vi "SetTilesByString.vi"(8 "error in (no error)":errorcluster, 9 "Position":T1, 10 "TileStrings":string[][](array[string]), 11 "TilesQueue":refnum<queue>) -> (0 "error out":errorcluster, 3 "TilesQueue out":refnum<queue>)   [LabVIEW 2019, in "RT_Game.lvlib" / "Engine.lvclass"]
uses:
  Engine.lvclass
  Game/Coordinate.ctl
  MessageCluster.ctl
  SetTilesByStringData.ctl
  Game/Game.lvclass
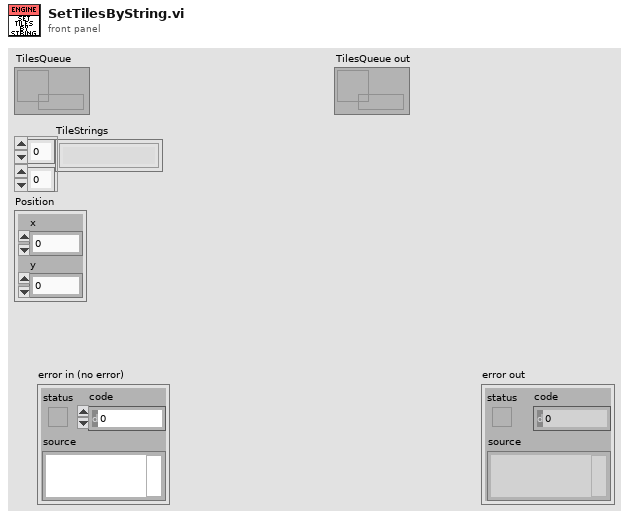
[diagram p1: front panel]
types:
  T1 = typedef "RT_Game.lvlib/Game.lvclass/Coordinate.ctl" = cluster{"x":dbl, "y":dbl}
  T2 = typedef "RT_Game.lvlib/Engine.lvclass/MessageCluster.ctl" = cluster{"Message":string, "Data":variant}
  T3 = typedef "RT_Game.lvlib/Engine.lvclass/SetTilesByStringData.ctl" = cluster{"TileStrings":string[][], "Position":T1}
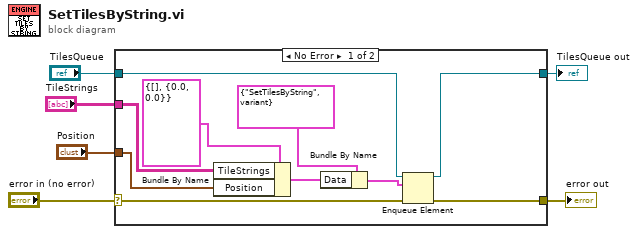
[diagram p0: block diagram]
diagram:
  n1 = case shown="No Error" "error in (no error)" {
    selector: "error in (no error)" -> [w11 w18]
    tunnel: [w12 w18] -> w5
    tunnel: "TileStrings" -> [w10 _]
    tunnel: "Position" -> [w9 _]
    tunnel: "TilesQueue" -> [w8 w17]
    tunnel: [w7 w17] -> w1
    frame No Error {
      n2 = Bundle By Name(cluster=T3 {"TileStrings"=[], "Position"={"x"=0.0, "y"=0.0}} ("SetTilesByStringData"), "TileStrings"=w10, "Position"=w9) -> (w16:T3)
      n3 = Bundle By Name(cluster=T2 {"Message"="SetTilesByString", "Data"=variant} ("element"), "Data"=w16) -> (w14:T2)
      n4 = Enqueue Element(queue=w8, element=w14, error in (no error)=w11) -> (queue out=w7:refnum<queue>, error out=w12:errorcluster)  [unwired: 1 in, 1 out]
    }
    frame Error {
    }
  }
  "error out" <- w5
  "TilesQueue out" <- w1
